vi "SIAMScript_to_String.vi"(8 "error in (no error)":errorcluster, 11 "Script":T2(array[cluster])=[{"Delay 10µs"=0, "command"=4027514895, "P0"=16777215, "P1"=0, "P2"=0, "P3"=0, "P4"=0, "P5-ticket"=0, "comment"=""}, {"Delay 10µs"=0, "command"=4027514895, "P0"=100, "P1"=0, "P2"=0, "P3"=0, "P4"=0, "P5-ticket"=0, "comment"=""}, {"Delay 10µs"=0, "command"=4027514895, "P0"=5, "P1"=120, "P2"=0, "P3"=0, "P4"=0, "P5-ticket"=0, "comment"=""}] {"command" format="%x" items=["end_no_ticket"=4027514895, "end_ticket"=4027518991, "NoOp"=4026531840, "Read ticks"=4026535936, "Read ticks to var"=4026535938, "Read IP"=4043313152, "Read IP into var"=4043313154, "Set IP from var"=4043309059, "Set IP from var, relative"=4043313155, "branchRel_if_equal"=4043374849, "decrement_branchRel_if_equal"=4043374945, "decrement_branchRel_if_greaterequal"=4043375201, "decrement_branchRel_if_greaterequal_withTicket"=4043379297, "decrement_branchRel_if_smaller"=4043375457, "increment_branchRel_if_smaller"=4043375473, "readVar"=4060090368, "writeVar"=4060086273, "copyVar0_from_var1"=4060086275, "math_addToVariable"=4076863488, "math_addVToVariable"=4076863489, "math_subToVariable"=4076863490, "math_subVToVariable"=4076863491, "math_multToVariable"=4076863492, "math_multvToVariable"=4076863493, "math_divideToVariable"=4076863494, "math_divideVToVariable"=4076863495, "math_modToVariable"=4076863496, "math_modVToVariable"=4076863497, "logic_and"=4093640704, "logic_or"=4093640706, "logic_xor"=4093640708, "bitshift"=4093640712, "I2C-write"=335544337, "I2C-read"=335548433, "Cam-SPI-write"=3254779905, "UART0-VC-Baud-write"=469958673, "UART0-VC-Baud-read"=469962768, "UART0-VC-write"=469762065, "UART0-VC-write-Var"=469762067, "UART0-VC-read-availabe-bytes-to-var"=470355970, "UART0-VC-read-availabe-bytes"=470355984, "UART0-VC-read-skip-bytes"=469831681, "UART0-VC-read"=469766160, "UART0-VC-read-Var"=469766162, "UART1-TSM-Baud-write"=486735889, "UART1-TSM-Baud-read"=486739984, "UART1-TSM-write"=486539281, "UART1-TSM-write-Var"=486539283, "UART1-TSM-read-availabe-bytes-to-var"=487133186, "UART1-TSM-read-availabe-bytes"=487133200, "UART1-TSM-read-skip-bytes"=486604801, "UART1-TSM-read-skip-bytes"=486608897, "UART1-TSM-read"=486543376, "UART1-TSM-read-Var"=486543378, "UART2-Laser-Baud-write"=503513105, "UART2-Baud-read"=503517200, "UART2-write"=503316497, "UART2-write-Var"=503316499, "UART2-read-availabe-bytes-to-var"=503910402, "UART2-read-availabe-bytes"=503910416, "UART2-read-skip-bytes"=503386113, "UART2-read"=503320592, "UART2-read-Var"=503320594, "UART3-Baud-write"=520290321, "UART3-Baud-read"=520294416, "UART3-write"=520093713, "UART3-write-Var"=520093715, "UART3-read-availabe-bytes-to-var"=520687618, "UART3-read-availabe-bytes"=520687632, "UART3-read-skip-bytes"=520163329, "UART3-read"=520097808, "UART3-read-Var"=520097810, "IO-read_bank0"=3489665024, "IO-write_bank0"=3489660929, "IO-read_bank1"=3506442240, "IO-write_bank1"=3506438145, "DA0-0_LED365"=2684354561, "DA0-1_LED385"=2685403137, "DA0-2_LED440"=2686451713, "DA0-3_LED470"=2687500289, "DA0-4_LED510"=2688548865, "DA0-5_LED550"=2689597441, "DA0-6_LED590"=2690646017, "DA0-7_LED640"=2691694593, "DA1-0_LED-R"=2701131777, "DA1-1_LED-G"=2702180353, "DA1-2_LED-B"=2703228929, "DA1-3_LED-AF"=2704277505, "DA1-4"=2705326081, "DA1-5"=2706374657, "DA1-6"=2707423233, "DA1-7"=2708471809, "DA2-Laser0"=2717908993, "DA2-Laser1"=2718957569, "DA2-Laser2"=2720006145, "DA2-Laser3"=2721054721, "DA2-Laser4"=2722103297, "Analog-read_AD0-0"=2818576384, "Analog-read-store_AD0-0"=2818572290, "AF-Register-transfer r/w"=2835349505, "AF-Register-read"=2835353600, "AF-Register-read-to-var"=2835353602, "AF-Transfer-from-var"=2835349507, "IO-delay_bank0"=3489923073, "IO-delay_bank0_fromVar"=3489923075, "read_cam_clock"=3289124864, "store_cam_clock"=3289120770, "read_cam_phase"=3289190400, "store_cam_phase"=3289186306, "store_cam_phase-t"=3289190402, "r_cam1_NHS"=3254980608, "w_cam1_NHS"=3254976513, "r_cam1_NVS"=3255046144, "w_cam1_NVS"=3255042049, "r_cam1_npx"=3255111680, "w_cam1_npx"=3255107585, "r_cam1_npy"=3255177216, "w_cam1_npy"=3255173121, "r_cam1_xhswait"=3255439360, "w_cam1_xhswait"=3255435265, "r_cam1_xvs_wait"=3255504896, "w_cam1_xvs_wait"=3255500801, "r_cam1_framcounter"=3255570432, "r_cam1_line"=3255635968, "r_cam1_xhs-counter"=3255701504, "r_cam2_NHS"=3271757824, "w_cam2_NHS"=3271753729, "r_cam2_NVS"=3271823360, "w_cam2_NVS"=3271819265, "r_cam2_npx"=3271888896, "w_cam2_npx"=3271884801, "r_cam2_npy"=3271954432, "w_cam2_npy"=3271950337, "r_cam2_xvs_wait"=3272282112, "w_cam2_xvs_wait"=3272278017, "r_cam2_framcounter"=3272347648, "r_cam2_line"=3272413184, "r_cam2_xhs-counter"=3272478720, "start TMSI"=102694919, "set_1Galvo"=101712113, "set_x-Galvo"=102760689, "set_y-Galvo"=103809265, "set_z-Fokus"=104857841, "set_1Galvo_position-only"=101711937, "set_x-Galvo_position-only"=102760513, "set_y-Galvo_position-only"=103809089, "set_z-Fokus_position-only"=104857665, "set_x-Galvo_position-only_ticket"=102764609, "set_y-Galvo_position-only_ticket"=103813185, "set_z-Fokus_position-only_ticket"=104861761, "set_1Galvo_relativ-only"=101712001, "set_x-Galvo_relativ-only"=102760577, "set_y-Galvo_relativ-only"=103809153, "set_z-Fokus_relativ-only"=104857729, "set_1Galvo_speed-only"=101711905, "set_x-Galvo_speed-only"=102760481, "set_y-Galvo_speed-only"=103809057, "set_z-Fokus_speed-only"=104857633, "set_1Galvo_acc-only"=101711889, "set_x-Galvo_acc-only"=102760465, "set_y-Galvo_acc-only"=103809041, "set_z-Fokus_acc-only"=104857617, "read_1Galvo_ticket"=101716032, "read_x-Galvo_ticket"=102764608, "read_y-Galvo_ticket"=103813184, "read_z-Focus_ticket"=104861760, "x-Galvo_pos_fromVar"=102760515, "y-Galvo_pos_fromVar"=103809091, "z-Focus_pos_fromVar"=104857667, "Servo0"=67108865, "Servo0-enable"=68091911, "Servo0-disable"=68091919, "Servo1"=68157441, "Servo1-enable"=69140487, "Servo1-disable"=69140495, "Servo2-enable"=70189063, "Servo2"=69206017, "Servo3-enable"=71237639, "Servo3"=70254593, "x-ssi-init"=202309639, "x-ssi-disable"=202309647, "x-ssi-Bits"=201523201, "x-ssi-Read"=201330688, "x-ssi-ReadToVar"=201326594, "x-ssi-ReadToVar-ticket"=201330690, "y-ssi-init"=203358215, "y-ssi-disable"=203358223, "y-ssi-Bits"=202571777, "y-ssi-Read"=202379264, "y-ssi-ReadToVar"=202375170, "y-ssi-ReadToVat-ticket"=202379266]}) -> (0 "error out":errorcluster, 3 "String":string="00000000 0D000001 00FFFFFF 00000000 00000000 00000000 00000000 00000100\n00000000 C40A0001 00000064 00000000 00000000 00000000 00000000 00000101\n00000000 F2000001 00000057 00000078 00000000 00000000 00000000 00000102\n00000000 C40B0003 00000057 00000000 00000000 00000000 00000000 00000103\n00000001 C40F000A 00000000 00000000 00000000 00000000 00000000 00000104\n00000000 C40C1000 00000000 00000000 00000000 00000000 00000000 00000105\n00000000 C40D1000 00000000 00000000 00000000 00000000 00000000 00000106\n00000000 C40E0002 00000056 00000000 00000000 00000000 00000000 00000107\n00000000 F2000006 00000056 FFFFFFCE 00000000 00000000 00000000 00000108\n00000000 0D041003 00000056 00000000 00000000 00000000 00000000 00000109\n00000001 F1011261 00000000 00000057 00000002 00000000 00000000 0000010A\n00000000 0D000001 00000001 00000001 00000000 00000000 00000000 0000010B\n00000002 0D000001 00000001 00000000 00000000 00000000 00000000 0000010C\n00000001 F00F100F 00000000 00000000 00000000 00000000 00000000 00000FFF")   [LabVIEW 2011]
uses:
  SIAM_command.ctl
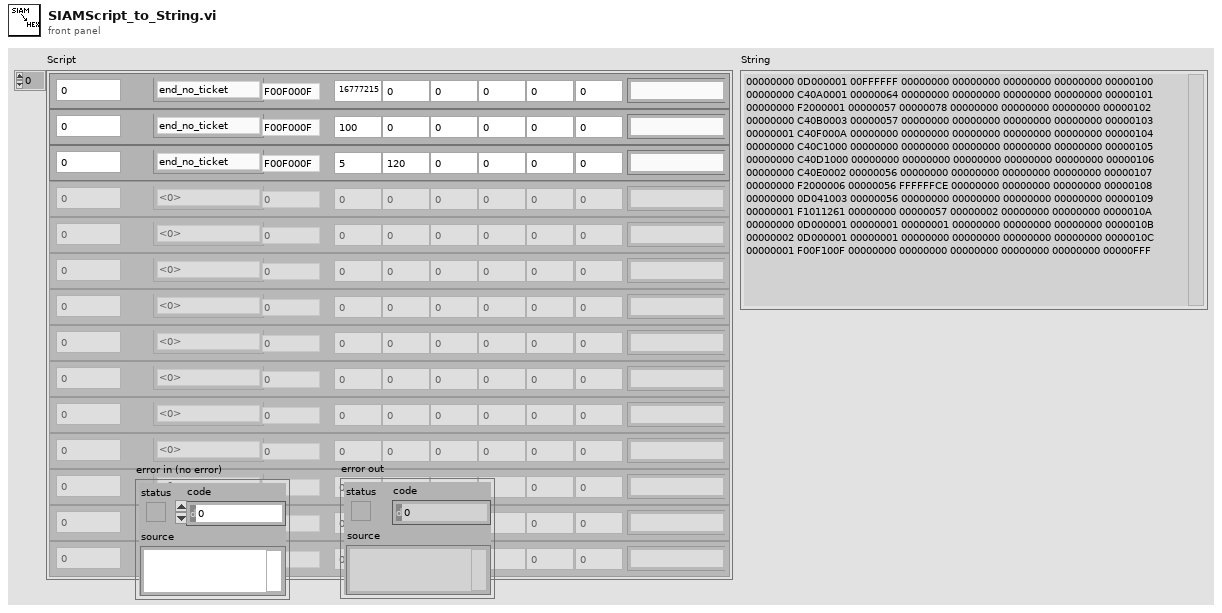
[diagram p1: front panel]
types:
  T1 = typedef "SIAM_command.ctl" = u32
  T2 = cluster{"Delay 10µs":u32, "command":T1, "P0":i32, "P1":i32, "P2":i32, "P3":i32, "P4":i32, "P5-ticket":i32, "comment":string}[]
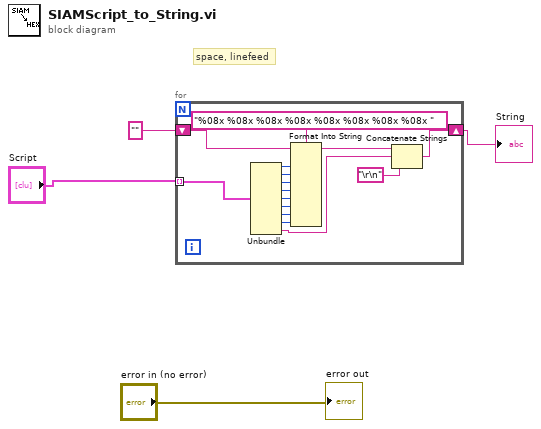
[diagram p0: block diagram]
diagram:
  # "space, linefeed"
  n1 = for {
    tunnel: "Script" -> [w19] mode=indexing
    shift-right: [w7] -> w1
    shift-left: "" -> [w8]
    n2 = Unbundle(w19) -> ("Delay 10µs"=w18:u32, "command"=w17:T1, "P0"=w16:i32, "P1"=w15:i32, "P2"=w14:i32, "P3"=w13:i32, "P4"=w12:i32, "P5-ticket"=w11:i32, "comment"=w6:string)
    n3 = Format Into String(format string="%08x %08x %08x %08x %08x %08x %08x %08x ", initial string=w8, w18, w17, w16, w15, w14, w13, w12, w11) -> (resulting string=w9:string)  [unwired: 1 in, 1 out]
    n4 = Concatenate Strings(w9, w6, "\r\n") -> (w7:string)
  }
  "String" <- w1
  "error out" <- "error in (no error)"
